vi "GameOver.vi"(8 "error in (no error)":errorcluster, 11 "Bouncer in":refnum<class "Bouncer.lvclass">) -> (0 "error out":errorcluster, 3 "Bouncer out":refnum<class "Bouncer.lvclass">)   [LabVIEW 2019, in "RT_Game.lvlib" / "Bouncer.lvclass"]
uses:
  Bouncer.lvclass
  C:/Users/FreshBob/Dropbox/VIs/myRIO_GameConsole/RT/RT_Game/Game/Game.lvclass
  Bouncer.lvclass/Bouncer.ctl
  Game/Coordinate.ctl
  BounceTarget/BounceTarget.lvclass/BounceTarget.ctl
  GameObject/GameObject.lvclass/GameObject.ctl
  BounceTarget/Write Lives.vi
  GameObject/Write IsActive.vi
  BounceTarget/Write DoDraw.vi
  BounceTarget/BounceTarget.lvclass
  C:/Users/FreshBob/Dropbox/VIs/myRIO_GameConsole/RT/RT_Game/GameObject/GameObject.lvclass
  PongBall/PongBall.lvclass
  Game/Game.lvclass
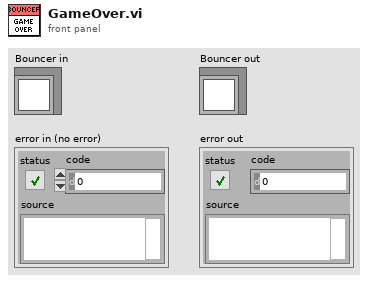
[diagram p1: front panel]
types:
  T1 = enum16{"all", "up", "down", "left", "right", "leftup", "rightup", "leftdown", "rightdown"}
  T2 = typedef "RT_Game.lvlib/Game.lvclass/Coordinate.ctl" = cluster{"x":dbl, "y":dbl}
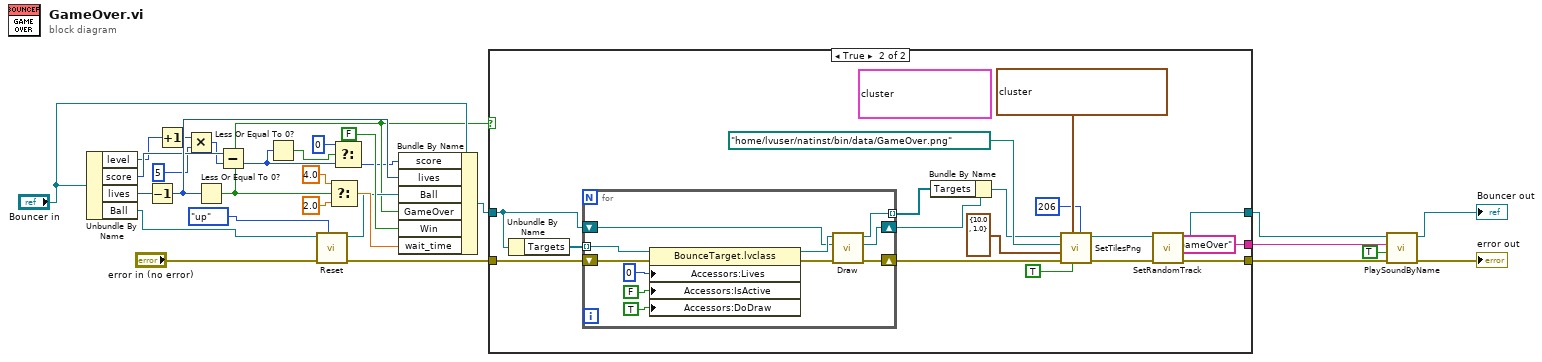
[diagram p0: block diagram]
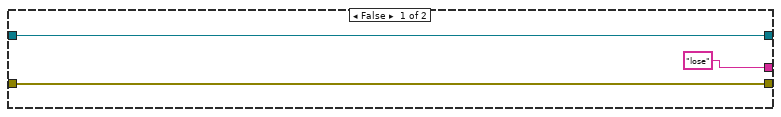
[diagram p2: hidden frame]
diagram:
  n1 = Unbundle By Name("Bouncer in") -> ("level"=w3:i16, "score"=w14:i16, "lives"=w24:i16, "Ball"=w22:refnum<class "PongBall.lvclass">)
  n2 = Decrement(x=w24) -> (x-1=w25:i16)
  n3 = Increment(x=w3) -> (x+1=w1:i16)
  n4 = Multiply(x=w1, y=i16 5 ("x")) -> (x*y=w2:i16)
  n5 = Less Or Equal To 0?(x=w25) -> (x <= 0?=w15:bool)
  n6 = Subtract(x=w14, y=w2) -> (x-y=w11:i16)
  n7 = Less Or Equal To 0?(x=w11) -> (x <= 0?=w10:bool)
  n8 = call "Reset.vi"("Direction (all)"=T1."up", "error in (no error)"="error in (no error)", "PongBall in"=w22) -> ("error out"=w21:errorcluster, "PongBall out"=w23:refnum<class "PongBall.lvclass">)  [unwired: 7 in]
  n9 = Select(t=4.0, s=w15, f=2.0 ("wait_time")) -> (s? t:f=w28:dbl)
  n10 = Select(t=i16 0, s=w10, f=w11) -> (s? t:f=w13:i16)
  n11 = Bundle By Name(cluster="Bouncer in", "score"=w13, "lives"=w25, "Ball"=w23, "GameOver"=w15, "Win"=FALSE, "wait_time"=w28) -> (w16:refnum<class "Bouncer.lvclass">)
  n12 = case shown="True" w15 {
    tunnel: w21 -> [w31 w42]
    tunnel: [w31 w38] -> w17
    tunnel: w16 -> [w32 w43]
    tunnel: [w32 w36] -> w7
    tunnel: ["lose" ("Name") "GameOver" ("Name")] -> w6
    frame False {
    }
    frame True {
      (unwired) cluster{"Color":fxp<+,3,3>, "TileCode":string}[] [{"Color"=0.0, "TileCode"="XX#replace-0-1"}] ("Tiles")
      n13 = Unbundle By Name(w43) -> ("Targets"=w46:refnum<class "BounceTarget.lvclass">[])
      n14 = for {
        tunnel: w46 -> [w58] mode=indexing
        tunnel: [w54] -> w45 mode=indexing
        shift-right: [w56] -> w41
        shift-left: w42 -> [w60]
        shift-right: [w52] -> w44
        shift-left: w43 -> [w53]
        n15 = property class="BounceTarget.lvclass"(reference=w58, error in=w60, "Accessors:Lives"=i16 0 ("Lives"), "Accessors:IsActive"=FALSE ("IsActive"), "Accessors:DoDraw"=TRUE ("DoDraw")) -> (reference out=w55:refnum<class "BounceTarget.lvclass">, error out=w59:errorcluster)
        n16 = call "Draw.vi"("error in (no error)"=w59, "RT_Game.lvlib:Game.lvclass"=w53, "BounceTarget in"=w55) -> ("error out"=w56:errorcluster, "RT_Game.lvlib:Game.lvclass 2"=w52:refnum<class "Bouncer.lvclass">, "BounceTarget out"=w54:refnum<class "BounceTarget.lvclass">)  [unwired: 6 in]
      }
      n17 = Bundle By Name(cluster=w44, "Targets"=w45) -> (w40:refnum<class "Bouncer.lvclass">)
      n18 = call "SetTilesPng.vi"("DefaultTileCode"=u32 206, "Draw (true)"=TRUE, "Tiles"=cluster{"Color":fxp<+,3,3>, "TileCode":u32}[] [{"Color"=0.0, "TileCode"=536871118}], "error in (no error)"=w41, "Position"=T2 {"x"=10.0, "y"=1.0}, "Path"=path "/home/lvuser/natinst/bin/data/GameOver.png", "Game in"=w40) -> ("error out"=w39:errorcluster, "Game out"=w37:refnum<class "Bouncer.lvclass">)  [unwired: 1 in, 2 out]
      n19 = call "SetRandomTrack.vi"("error in (no error)"=w39, "Game in"=w37) -> ("error out"=w38:errorcluster, "Game out"=w36:refnum<class "Bouncer.lvclass">)  [unwired: 8 in]
    }
  }
  n20 = call "PlaySoundByName.vi"("error in (no error)"=w17, "Overwrite"=TRUE, "Name"=w6, "Game in"=w7) -> ("error out"=→"error out":errorcluster, "Game out"=→"Bouncer out":refnum<class "Bouncer.lvclass">)  [unwired: 6 in]
